vi "JH z-slider motor fixed step counter.vi"(5 "Number of steps":u16=2000, 6 "arrow presses":u16=1, 7 "Direction":enum16{"X +", "X -", "Y +", "Y -", "Z +", "Z -"}(ring)=enum."Z -", 8 "Error in (no error)":errorcluster, 9 "Amplitude (V) (NaN=no change)":sgl=nan, 10 "Frequency (Hz) (NaN=no change)":sgl=nan, 11 "Application ref in":refnum<vi>) -> (0 "Error out":errorcluster, 3 "Application ref out":refnum<vi>, 4 "press counter":i32)   [LabVIEW 2014]
uses:
  <userlib>/Nanonis Prog Interface V5/Nanonis Prog Interface.lvlib
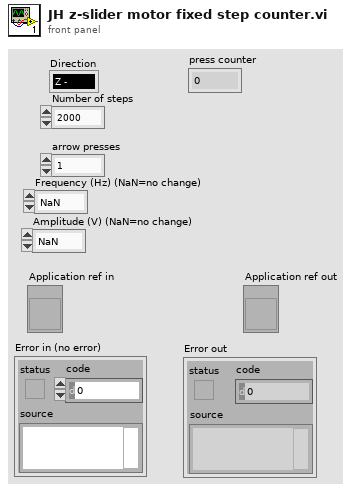
[diagram p1: front panel]
types:
  T1 = enum8{"Group 1", "Group 2", "Group 3", "Group 4", "Group 5", "Group 6"}
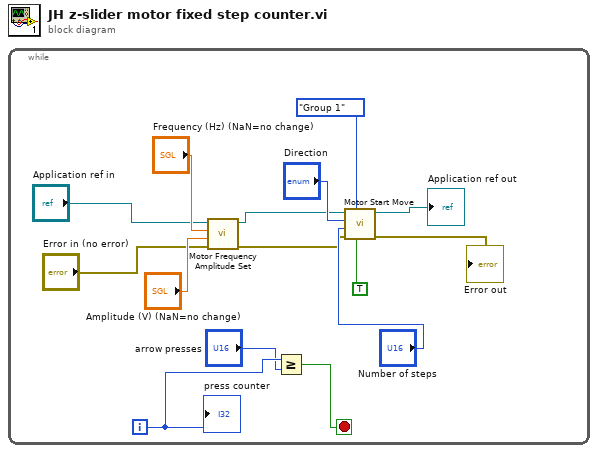
[diagram p0: block diagram]
diagram:
  n1 = while {
    i -> [w11]
    stop <- w9 stop-if-true
    n2 = call <userlib>:"Motor Frequency Amplitude Set.vi"("Error in (no error)"="Error in (no error)", "Amplitude (V) (NaN=no change)"="Amplitude (V) (NaN=no change)", "Frequency (Hz) (NaN=no change)"="Frequency (Hz) (NaN=no change)", "Application ref in"="Application ref in") -> ("Error out"=w7:errorcluster, "Application ref out"=w8:refnum<vi>)  [unwired: 6 in]
    n3 = Greater Or Equal?(x=w11, y="arrow presses") -> (x >= y?=w9:bool)
    n4 = call <userlib>:"Motor Start Move.vi"("Wait until finished? (F)"=TRUE, "Group"=T1."Group 1", "Error in (no error)"=w7, "Number of steps"="Number of steps", "Direction"="Direction", "Application ref in"=w8) -> ("Error out"=→"Error out":errorcluster, "Application ref out"=→"Application ref out":refnum<vi>)  [unwired: 3 in]
    "press counter" <- w11
  }
